vi "Main.vi"(8 "error in":errorcluster, 11 "Pumps Worker in":refnum<class "Pumps Worker.lvclass">) -> (0 "error out":errorcluster, 3 "Pumps Worker out":refnum<class "Pumps Worker.lvclass">)   [LabVIEW 2023, in "pump_Lib.lvlib" / "Pumps Worker.lvclass"]
doc: "The <b>Queued Message Handler</b> of the Worker that owns this VI."
uses:
  Pumps Worker.lvclass
  C:/Program Files/National Instruments/LabVIEW 2023/vi.lib/addons/_Workers/Library/Classes/Worker/Worker.lvclass
  TypeDef/control_Type.ctl
  TypeDef/pump_Type.ctl
  TypeDef/pair_Type.ctl
  Initialization Data.ctl
  Response Cases.ctl
  <vilib>/addons/_Workers/Library/Case Label.ctl
  Pumps Worker.lvclass/Pumps Worker.ctl
  rqp_Stop Session.ctl
  rqp_Get Settings.ctl
  rqp_Write Data.ctl
  TypeDef/pump_Type_Pair_L.ctl
  TypeDef/pump_Type_Pair_R.ctl
  rsp_New Pumps Data.ctl
  <vilib>/Utility/error.llb/Error Cluster From Error Code.vi
  <vilib>/ErrorRing/Error Ring.xnode
  <vilib>/addons/_Workers/Library/Classes/Message Queue/Message Queue.lvclass
  pump_Lib.lvlib
  Workers/Message Pump/Message Pump.lvclass
  <vilib>/addons/_Workers/Library/Workers.lvlib
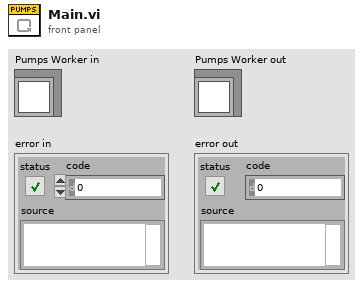
[diagram p1: front panel]
types:
  T1 = typedef "pump_Lib.lvlib/control_Type.ctl" = cluster{"IP Adress in":string, "control_Port_1 ref":refnum<vi>, "control_Port_2 ref":refnum<vi>, "control_Pair ref":refnum<vi>, "queue_Port 1":refnum<queue>, "queue_Port 2":refnum<queue>, "queue_Pair":refnum<queue>, "parametrs ref":refnum<vi>, "Stop Event":refnum<user-event>}
  T2 = typedef "pump_Lib.lvlib/Pumps Worker.lvclass/Initialization Data.ctl" = cluster{"Response Cases":T3}
  T3 = typedef "pump_Lib.lvlib/Pumps Worker.lvclass/Response Cases.ctl" = cluster{"Placeholder - Can be deleted":string, "New Pumps Data":T4}
  T4 = typedef "Workers.lvlib/Case Label.ctl" = string
  T5 = typedef "pump_Lib.lvlib/Pumps Worker.lvclass/rqp_Stop Session.ctl" = cluster{"String":string}
  T6 = typedef "pump_Lib.lvlib/Pumps Worker.lvclass/rqp_Get Settings.ctl" = cluster{"Pump":refnum<vi>, "Params":refnum<vi>, "Pump2":refnum<vi>, "Pump System":refnum<vi>, "IP Adress":string}
  T7 = typedef "pump_Lib.lvlib/Pumps Worker.lvclass/rqp_Write Data.ctl" = cluster{"Насос":T8, "Насос 2":T9, "Насосная система":T10}
  T8 = typedef "pump_Lib.lvlib/pump_Type_Pair_L.ctl" = cluster{"Давление заданное":dbl, "Давление MAX заданное":dbl, "Давление в насосе":dbl, "Давление в системе":dbl, "Расход заданый":dbl, "Расход текущий":dbl, "Объём заданный":dbl, "Объём текущий":dbl, "Позиция насоса %":dbl, "Ток двигателя":dbl, "controlMsg":string, "Клапан k_sys":bool, "Клапан k_res":bool, "Клапан k_air":bool, "Вверх":bool, "Домой":bool, "Вниз":bool, "Старт расход":bool, "Старт давление":bool, "Сброс объёма":bool, "Сброс давления Рсис":bool, "Сброс давления Рнас":bool, "Bits":cluster{"plc_control":bool, "lag_control":bool, "mstop_control":bool, "st_home":bool, "error":bool, "mstart":bool, "pair":bool, "startQ":bool, "startP":bool, "volume_Stop":bool}}
  T9 = typedef "pump_Lib.lvlib/pump_Type_Pair_R.ctl" = cluster{"Давление заданное":dbl, "Давление MAX заданное":dbl, "Давление в насосе":dbl, "Давление в системе":dbl, "Расход заданый":dbl, "Расход текущий":dbl, "Объём заданный":dbl, "Объём текущий":dbl, "Позиция насоса %":dbl, "Ток двигателя":dbl, "controlMsg":string, "Клапан k_sys":bool, "Клапан k_res":bool, "Клапан k_air":bool, "Вверх":bool, "Домой":bool, "Вниз":bool, "Старт расход":bool, "Старт давление":bool, "Сброс объёма":bool, "Сброс давления Рсис":bool, "Сброс давления Рнас":bool, "Bits":cluster{"plc_control":bool, "lag_control":bool, "mstop_control":bool, "st_home":bool, "error":bool, "mstart":bool, "pair":bool, "startQ":bool, "startP":bool, "volume_Stop":bool}}
  T10 = typedef "pump_Lib.lvlib/pair_Type.ctl" = cluster{"Давление заданное":dbl, "Давление в системе":dbl, "Расход заданый":dbl, "Расход текущий":dbl, "Объём заданный":dbl, "Объём текущий":dbl, "Старт давление":bool, "Старт расход":bool, "Сброс объёма":bool, "plc_control":bool, "lag_control":bool, "mstop_control":bool, "Давление":cluster{"АЦП CH 0":dbl, "АЦП CH 1":dbl, "АЦП CH 2":dbl, "АЦП CH 3":dbl, "АЦП CH 4":dbl, "АЦП CH 5":dbl, "АЦП CH 6":dbl, "АЦП CH 7":dbl}, "Modbus":cluster{"Массив чтения":u16[], "Массив записи":u16[]}}
  T11 = typedef "pump_Lib.lvlib/Pumps Worker.lvclass/rsp_New Pumps Data.ctl" = cluster{"Насос":T8, "Насос 2":T9, "Насосная система":T10}
  T12 = typedef "pump_Lib.lvlib/pump_Type.ctl" = cluster{"Давление заданное":dbl, "Давление MAX заданное":dbl, "Давление в насосе":dbl, "Давление в системе":dbl, "Расход заданый":dbl, "Расход текущий":dbl, "Объём заданный":dbl, "Объём текущий":dbl, "Позиция насоса %":dbl, "Ток двигателя":dbl, "controlMsg":string, "Клапан k_sys":bool, "Клапан k_res":bool, "Клапан k_air":bool, "Вверх":bool, "Домой":bool, "Вниз":bool, "Старт расход":bool, "Старт давление":bool, "Сброс объёма":bool, "Сброс давления Рсис":bool, "Сброс давления Рнас":bool, "Bits":cluster{"plc_control":bool, "lag_control":bool, "mstop_control":bool, "st_home":bool, "error":bool, "mstart":bool, "pair":bool, "startQ":bool, "startP":bool, "volume_Stop":bool}}
  T13 = cluster{"IP Adress in":string, "control_Port_1 ref":refnum<vi>, "control_Port_2 ref":refnum<vi>, "control_Pair ref":refnum<vi>, "queue_Port 1":refnum<queue>, "queue_Port 2":refnum<queue>, "queue_Pair":refnum<queue>, "parametrs ref":refnum<vi>, "Stop Event":refnum<user-event>}
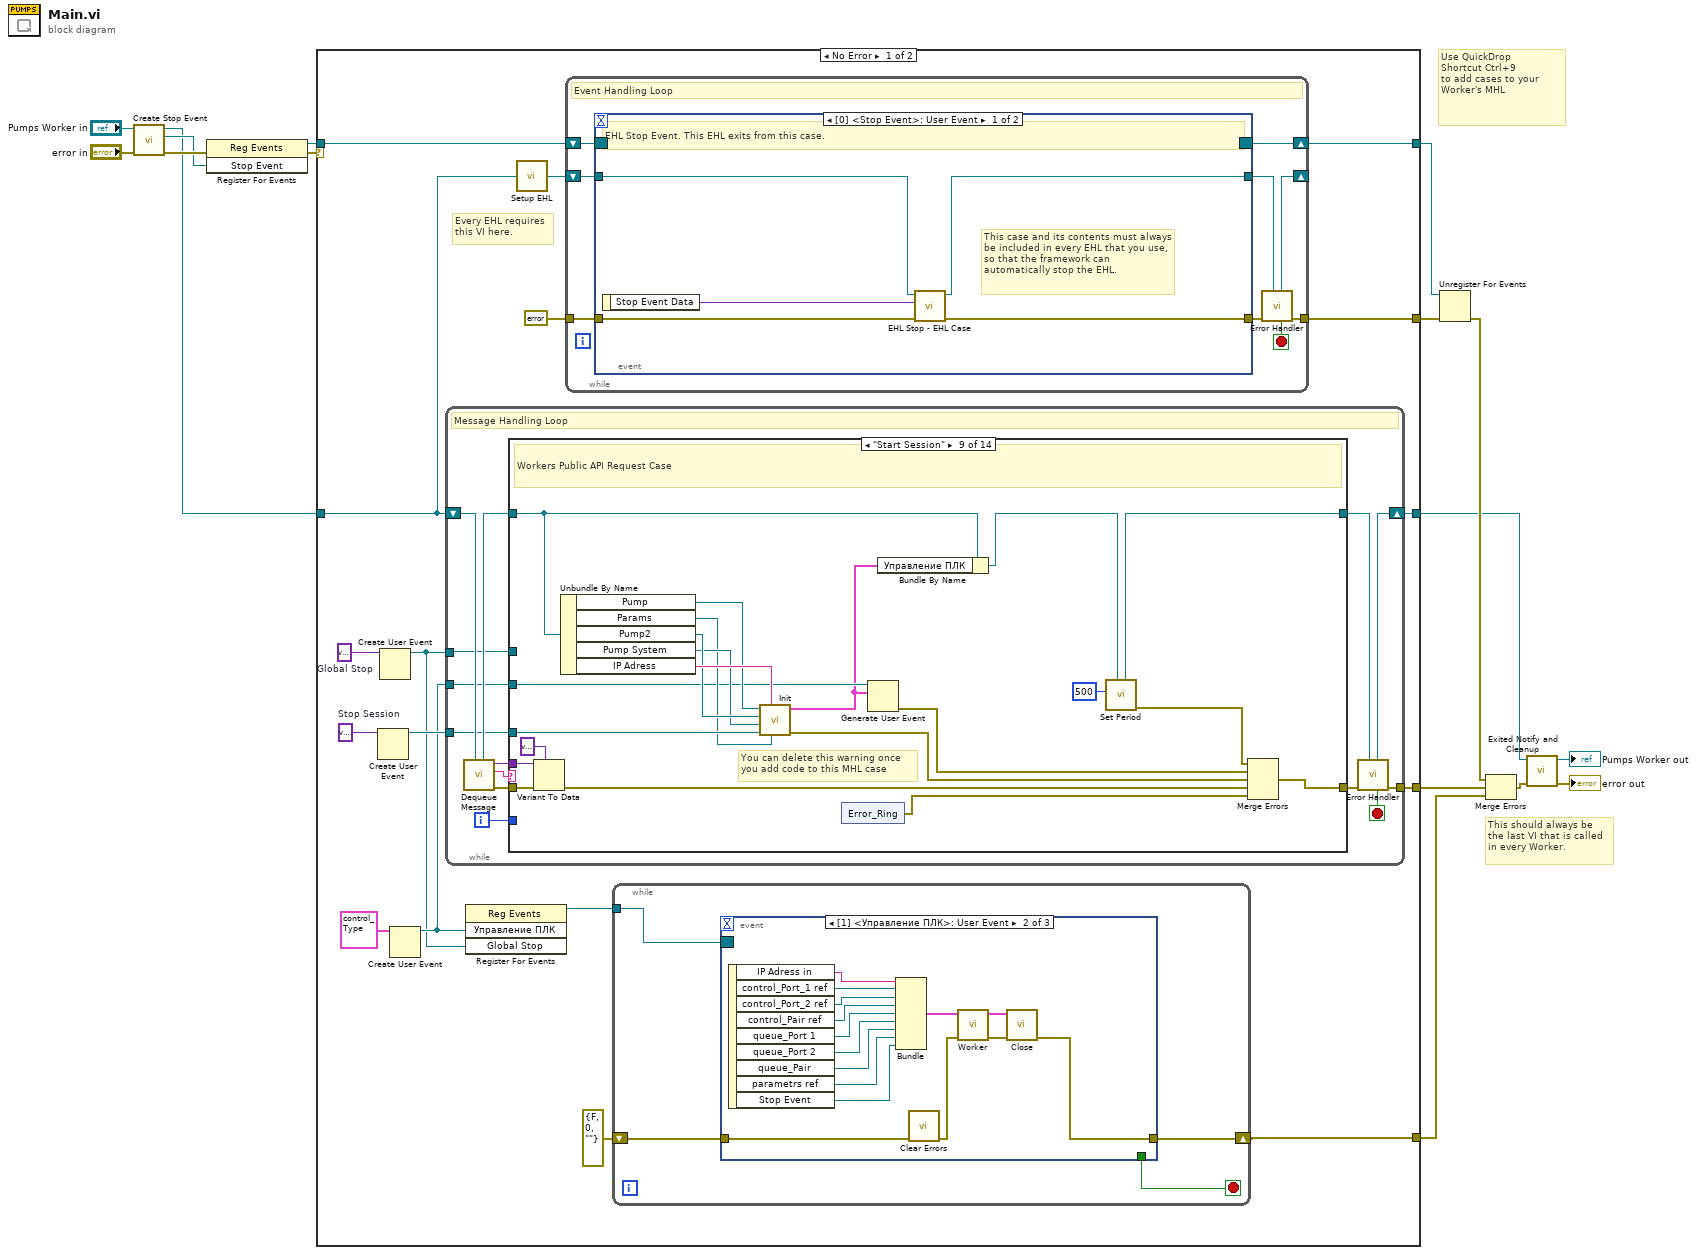
[diagram p0: block diagram]
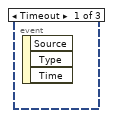
[diagram p2: hidden frame]
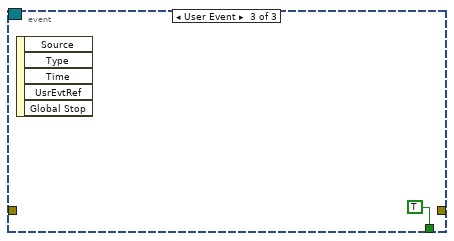
[diagram p3: hidden frame]
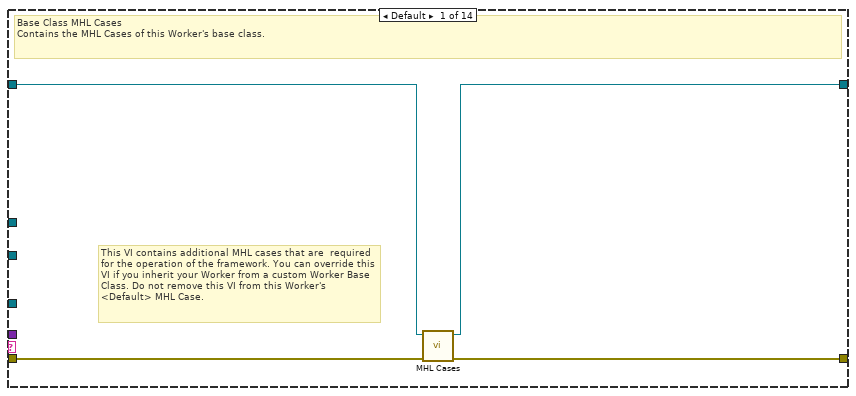
[diagram p4: hidden frame]
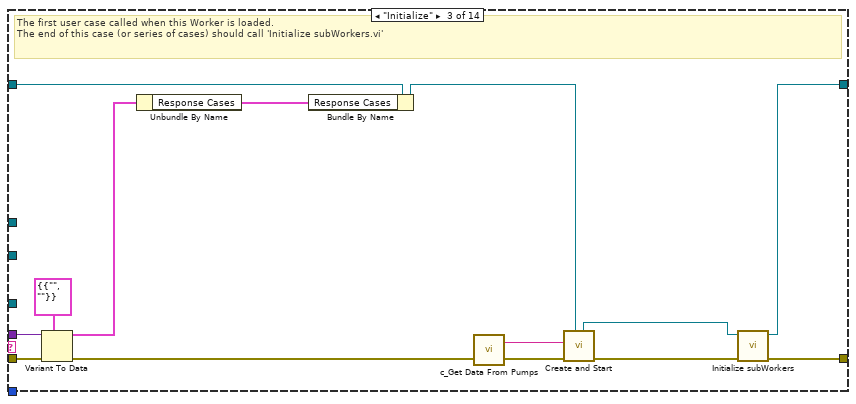
[diagram p6: hidden frame]
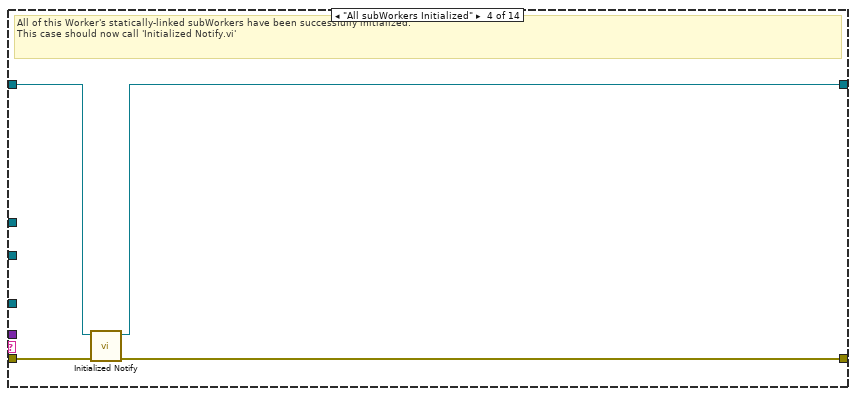
[diagram p7: hidden frame]
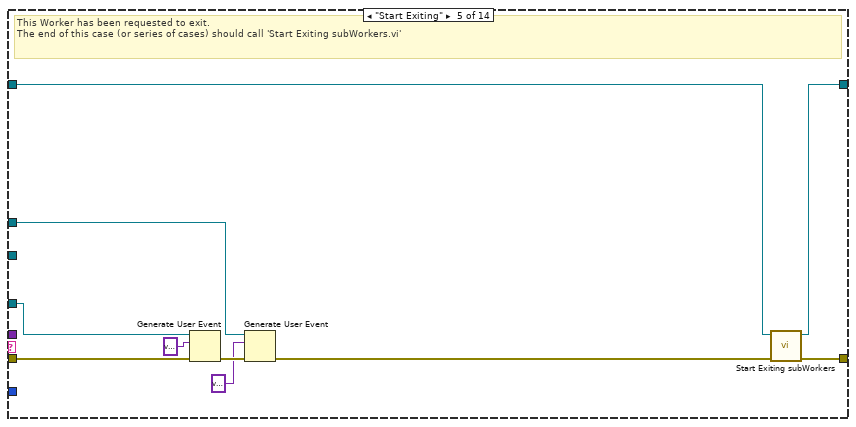
[diagram p8: hidden frame]
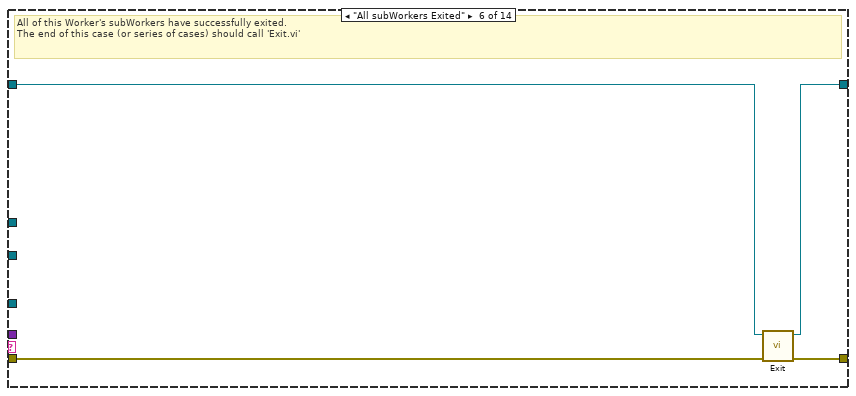
[diagram p9: hidden frame]
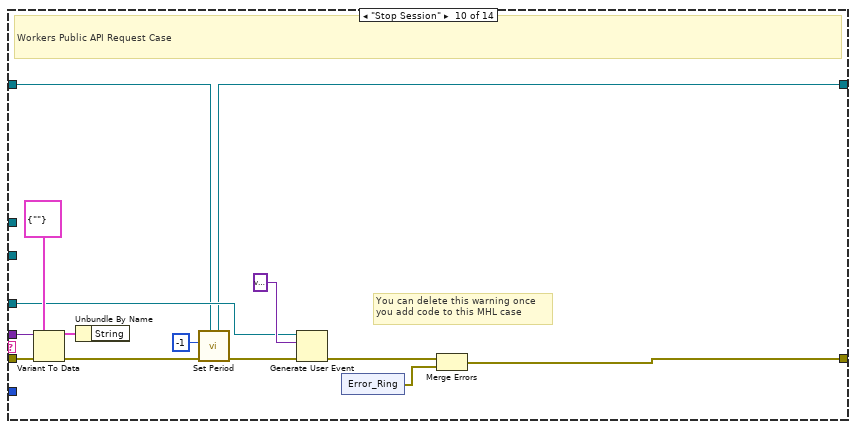
[diagram p12: hidden frame]
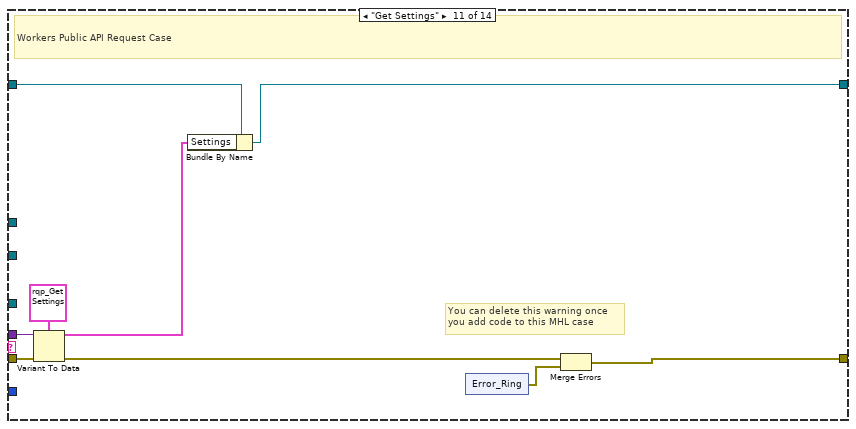
[diagram p13: hidden frame]
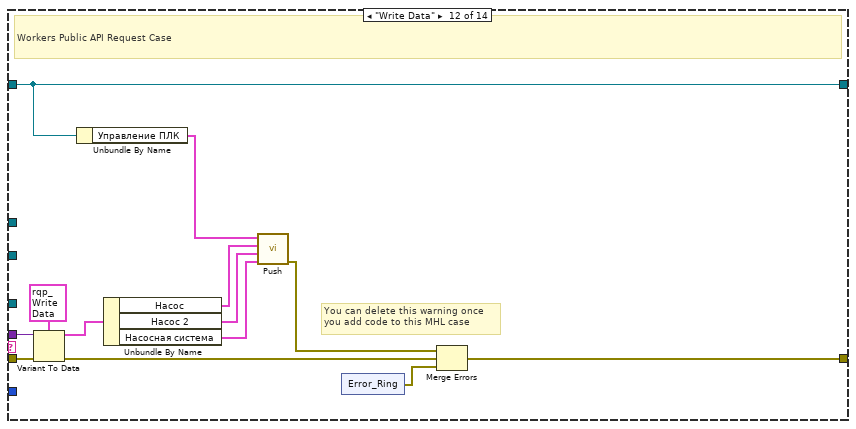
[diagram p14: hidden frame]
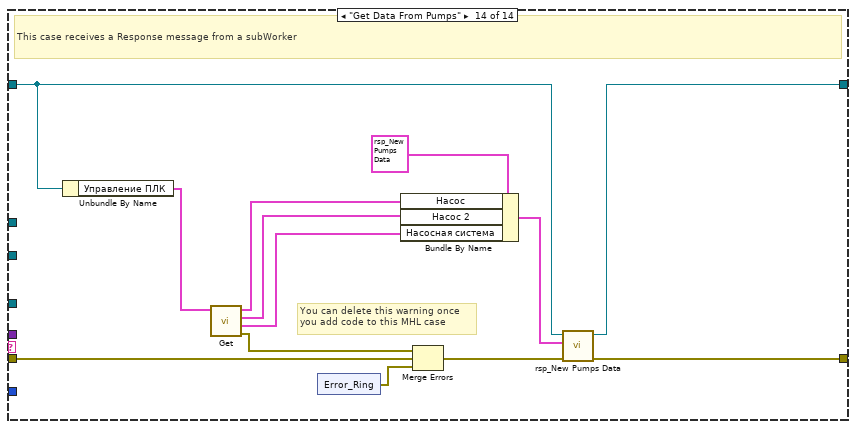
[diagram p16: hidden frame]
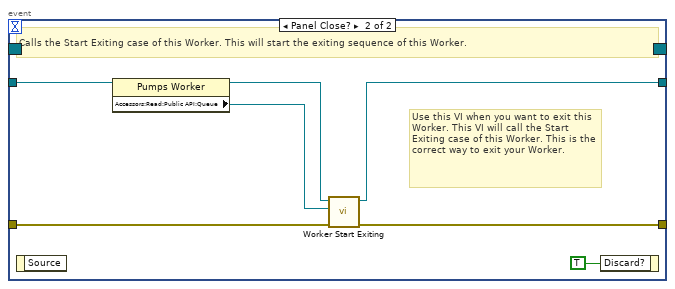
[diagram p17: hidden frame]
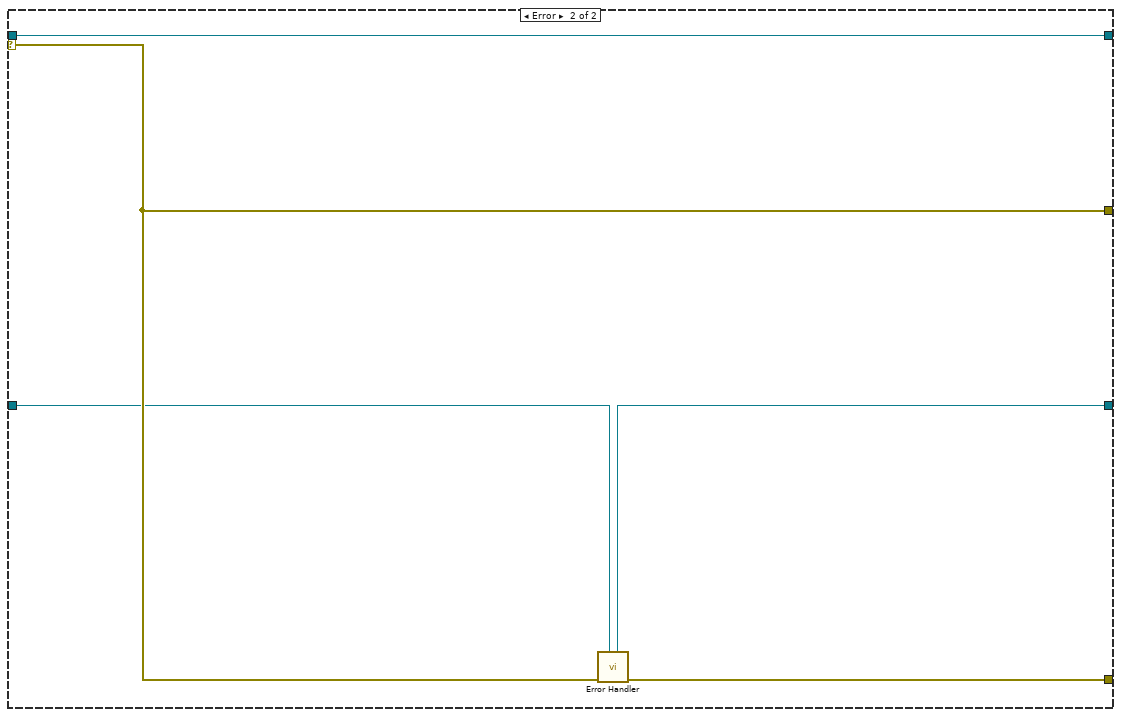
[diagram p18: hidden frame]
diagram:
  # "Use QuickDrop\nShortcut Ctrl+9\nto add cases to your\nWorker's MHL"
  # "This should always be the last VI that is called in every Worker."
  n1 = call-dynamic "Create Stop Event.vi"("error in"="error in", "Worker"="Pumps Worker in") -> ("error out"=w11:errorcluster, "Stop Event"=w8:refnum<user-event>, "Worker out"=w2:refnum<class "Pumps Worker.lvclass">)  [unwired: 7 in]
  n2 = register-events(error in=w11, w8) -> (reference out=w10:refnum<event-registration>, error out=w3:errorcluster)  [unwired: 1 in]
  n3 = case shown="No Error" w3 {
    tunnel: w2 -> [w28 w228]
    tunnel: [w26 w229] -> w9
    tunnel: w10 -> [w33 w230]
    tunnel: [w30 w231] -> w15
    tunnel: [w32 w230] -> w14
    tunnel: [w27 w227] -> w12
    selector: w3 -> [_ w231]
    tunnel: [w18 _] -> w1
    frame No Error {
      w20 = variant  # Global Stop
      w24 = variant  # Stop Session
      # "Every EHL requires\nthis VI here."
      n4 = Create User Event(user event datatype=w24) -> (user event=w23:refnum<user-event>)  [unwired: 1 in, 1 out]
      n5 = Create User Event(user event datatype=w20) -> (user event=w19:refnum<user-event>)  [unwired: 1 in, 1 out]
      n6 = Create User Event(user event datatype=T1 {"IP Adress in"="", "control_Port_1 ref"=refnum, "control_Port_2 ref"=refnum, "control_Pair ref"=refnum, "queue_Port 1"=refnum, "queue_Port 2"=refnum, "queue_Pair"=refnum, "parametrs ref"=refnum, "Stop Event"=refnum} ("Управление ПЛК")) -> (user event=w22:refnum<user-event>)  [unwired: 1 in, 1 out]
      n7 = while {
        shift-right: [w65] -> w27
        shift-left: w28 -> [w67]
        tunnel: [w66] -> w26
        tunnel: w22 -> [w57]
        tunnel: w23 -> [w56]
        tunnel: w19 -> [w54]
        i -> [w58]
        stop <- w59 stop-if-true
        # "Message Handling Loop"
        n8 = call-dynamic "Dequeue Message.vi"("Worker"=w67) -> ("error out"=w64:errorcluster, "Case out"=w60:string, "Data out"=w55:variant, "Worker out"=w62:refnum<class "Pumps Worker.lvclass">)  [unwired: 6 in, 1 out]
        n9 = case "Worker MHL Case Structure (DO NOT CHANGE LABEL NAME)" shown="\"Start Session\"" w60 {
          tunnel: w64 -> [w71 w72 w84 w88 w97 w104 w106 w108 w129 w148 w162 w180 w187 w200]
          tunnel: [w70 w72 w86 w87 w100 w103 w106 w108 w127 w144 w159 w175 w187 w193] -> w63
          tunnel: w62 -> [w69 w73 w83 w90 w98 w102 w105 w107 w115 w136 w157 w169 w186 w196]
          tunnel: [w68 w73 w85 w89 w99 w101 w105 w107 w111 w135 w155 w169 w186 w195] -> w61
          tunnel: w58 -> [_ _ _ _ _ _ _ _ _ _ _ _ _ _]
          tunnel: w57 -> [_ _ _ _ _ _ _ _ w117 _ _ _ _ _]
          tunnel: w56 -> [_ _ _ _ w96 _ _ _ w123 w137 _ _ _ _]
          tunnel: w55 -> [_ _ w82 _ _ _ _ _ w128 w146 w160 w177 _ _]
          tunnel: w54 -> [_ _ _ _ w92 _ _ _ _ _ _ _ _ _]
          frame Default {
            # "This VI contains additional MHL cases that are  required for the operation of the framework. You can override this VI if you inherit your Worker from a custom Worker Base Class. Do not remove this VI from this Worker's <Default> MHL Case."
            # "Base Class MHL Cases\nContains the MHL Cases of this Worker's base class."
            n10 = call-dynamic "MHL Cases.vi"("error in"=w71, "Worker in"=w69) -> ("error out"=w70:errorcluster, "Worker out"=w68:refnum<class "Pumps Worker.lvclass">)  [unwired: 8 in]
          }
          frame "------------ FRAMEWORK CASES -----------" {
            # "Start of Workers Framework Cases"
          }
          frame "Initialize" {
            # "The first user case called when this Worker is loaded.\nThe end of this case (or series of cases) should call 'Initialize subWorkers.vi'"
            n11 = Variant To Data(error in=w84, type=T2 {"Response Cases"={"Placeholder - Can be deleted"="", "New Pumps Data"=""}} ("Initialization Data"), Variant=w82) -> (data=w81:T2, error out=w75:errorcluster)
            n12 = Unbundle By Name(w81) -> ("Response Cases"=w80:T3)
            n13 = Bundle By Name(cluster=w83, "Response Cases"=w80) -> (w77:refnum<class "Pumps Worker.lvclass">)
            n14 = call "c_Get Data From Pumps.vi"() -> ("Case Label"=w78:T4)  [unwired: 1 in]
            n15 = call "Create and Start.vi"("Caller"=w77, "error in (no error)"=w75, "Time Elapsed Response Case (Case Label)"=w78) -> ("error out"=w74:errorcluster, "dup Caller out"=w76:refnum<class "Pumps Worker.lvclass">)  [unwired: 6 in, 1 out]
            n16 = call-dynamic "Initialize subWorkers.vi"("error in"=w74, "Worker"=w76) -> ("error out"=w86:errorcluster, "dup Worker out"=w85:refnum<class "Pumps Worker.lvclass">)  [unwired: 8 in]
          }
          frame "All subWorkers Initialized" {
            # "All of this Worker's statically-linked subWorkers have been successfully initialized.\nThis case should now call 'Initialized Notify.vi'"
            n17 = call-dynamic "Initialized Notify.vi"("error in"=w88, "Worker"=w90) -> ("error out"=w87:errorcluster, "dup Worker out"=w89:refnum<class "Pumps Worker.lvclass">)  [unwired: 8 in]
          }
          frame "Start Exiting" {
            # "This Worker has been requested to exit. \nThe end of this case (or series of cases) should call 'Start Exiting subWorkers.vi'"
            n18 = Generate User Event(user event=w96, event data cluster=variant ("event data"), error in=w97) -> (error out=w94:errorcluster)  [unwired: 1 in, 1 out]
            n19 = Generate User Event(user event=w92, event data cluster=variant ("event data"), error in=w94) -> (error out=w93:errorcluster)  [unwired: 1 in, 1 out]
            n20 = call-dynamic "Start Exiting subWorkers.vi"("error_in"=w93, "Worker"=w98) -> ("error out"=w100:errorcluster, "dup Worker out"=w99:refnum<class "Pumps Worker.lvclass">)  [unwired: 8 in]
          }
          frame "All subWorkers Exited" {
            # "All of this Worker's subWorkers have successfully exited. \nThe end of this case (or series of cases) should call 'Exit.vi'"
            n21 = call-dynamic "Exit.vi"("error_in"=w104, "Worker"=w102) -> ("error out"=w103:errorcluster, "dup Worker out"=w101:refnum<class "Pumps Worker.lvclass">)  [unwired: 8 in]
          }
          frame "------------- LOCAL API CASES -------------" {
            # "Start of Workers Local API Cases"
          }
          frame "------------- PUBLIC API CASES -------------" {
            # "Start of Workers Public API Cases"
          }
          frame "Start Session" {
            # "You can delete this warning once\nyou add code to this MHL case"
            # "Workers Public API Request Case"
            n22 = Variant To Data(error in=w129, type=variant, Variant=w128) -> (error out=w125:errorcluster)  [unwired: 1 out]
            n23 = Unbundle By Name(w115) -> ("Pump"=w121:refnum<vi>, "Params"=w118:refnum<vi>, "Pump2"=w120:refnum<vi>, "Pump System"=w119:refnum<vi>, "IP Adress"=w122:string)
            n24 = call "Init.vi"("parametrs ref"=w118, "IP Adress in"=w122, "Stop Event"=w123, "control_Pair ref"=w119, "control_Port_2 ref"=w120, "control_Port_1 ref"=w121) -> ("error out"=w124:errorcluster, "Управление ПЛК"=w114:T1)  [unwired: 4 in]
            n25 = xnode ("Error_Ring")() -> ("error out"=w126:errorcluster)
            n26 = Generate User Event(user event=w117, event data cluster=w114) -> (error out=w116:errorcluster)  [unwired: 2 in, 1 out]
            n27 = Bundle By Name(cluster=w115, "Управление ПЛК"=w114) -> (w112:refnum<class "Pumps Worker.lvclass">)
            n28 = call "Set Period.vi"("Caller"=w112, "Period (ms)"=500) -> ("error out"=w110:errorcluster, "dup Caller out"=w111:refnum<class "Pumps Worker.lvclass">)  [unwired: 8 in]
            n29 = Merge Errors(w110, w116, w124, w125, w126) -> (w127:errorcluster)
          }
          frame "Stop Session" {
            # "You can delete this warning once\nyou add code to this MHL case"
            # "Workers Public API Request Case"
            n30 = Variant To Data(error in=w148, type=T5 {"String"=""} ("Data"), Variant=w146) -> (data=w145:T5, error out=w139:errorcluster)
            n31 = Unbundle By Name(w145) -> ()  [unwired: 1 out]
            n32 = call "Set Period.vi"("Caller"=w136, "error in"=w139, "Period (ms)"=-1) -> ("error out"=w138:errorcluster, "dup Caller out"=w135:refnum<class "Pumps Worker.lvclass">)  [unwired: 7 in]
            n33 = Generate User Event(user event=w137, event data cluster=variant ("event data"), error in=w138) -> (error out=w142:errorcluster)  [unwired: 1 in, 1 out]
            n34 = xnode ("Error_Ring")() -> ("error out"=w143:errorcluster)
            n35 = Merge Errors(w142, w143) -> (w144:errorcluster)
          }
          frame "Get Settings" {
            # "You can delete this warning once\nyou add code to this MHL case"
            # "Workers Public API Request Case"
            n36 = Variant To Data(error in=w162, type=T6 {"Pump"=refnum, "Params"=refnum, "Pump2"=refnum, "Pump System"=refnum, "IP Adress"=""} ("Data"), Variant=w160) -> (data=w156:T6, error out=w154:errorcluster)
            n37 = Bundle By Name(cluster=w157, "Settings"=w156) -> (w155:refnum<class "Pumps Worker.lvclass">)
            n38 = xnode ("Error_Ring")() -> ("error out"=w158:errorcluster)
            n39 = Merge Errors(w154, w158) -> (w159:errorcluster)
          }
          frame "Write Data" {
            # "You can delete this warning once\nyou add code to this MHL case"
            # "Workers Public API Request Case"
            n40 = Variant To Data(error in=w180, type=T7 {"Насос"={"Давление заданное"=0.3, "Давление MAX заданное"=100.0, "Давление в насосе"=0.0, "Давление в системе"=99.99, "Расход заданый"=0.0, "Расход текущий"=0.0, "Объём заданный"=0.0, "Объём текущий"=0.0, "Позиция насоса %"=0.0, "Ток двигателя"=0.0, "controlMsg"="", "Клапан k_sys"=FALSE, "Клапан k_res"=FALSE, "Клапан k_air"=FALSE, "Вверх"=FALSE, "Домой"=FALSE, "Вниз"=FALSE, "Старт расход"=FALSE, "Старт давление"=FALSE, "Сброс объёма"=FALSE, "Сброс давления Рсис"=FALSE, "Сброс давления Рнас"=FALSE, "Bits"={"plc_control"=FALSE, "lag_control"=FALSE, "mstop_control"=FALSE, "st_home"=FALSE, "error"=FALSE, "mstart"=FALSE, "pair"=FALSE, "startQ"=FALSE, "startP"=FALSE, "volume_Stop"=FALSE}}, "Насос 2"={"Давление заданное"=0.3, "Давление MAX заданное"=100.0, "Давление в насосе"=0.0, "Давление в системе"=99.99, "Расход заданый"=0.0, "Расход текущий"=0.0, "Объём заданный"=0.0, "Объём текущий"=0.0, "Позиция насоса %"=0.0, "Ток двигателя"=0.0, "controlMsg"="", "Клапан k_sys"=FALSE, "Клапан k_res"=FALSE, "Клапан k_air"=FALSE, "Вверх"=FALSE, "Домой"=FALSE, "Вниз"=FALSE, "Старт расход"=FALSE, "Старт давление"=FALSE, "Сброс объёма"=FALSE, "Сброс давления Рсис"=FALSE, "Сброс давления Рнас"=FALSE, "Bits"={"plc_control"=FALSE, "lag_control"=FALSE, "mstop_control"=FALSE, "st_home"=FALSE, "error"=FALSE, "mstart"=FALSE, "pair"=FALSE, "startQ"=FALSE, "startP"=FALSE, "volume_Stop"=FALSE}}, "Насосная система"={"Давление заданное"=0.3, "Давление в системе"=99.99, "Расход заданый"=0.0, "Расход текущий"=0.0, "Объём заданный"=0.0, "Объём текущий"=0.0, "Старт давление"=FALSE, "Старт расход"=FALSE, "Сброс объёма"=FALSE, "plc_control"=FALSE, "lag_control"=FALSE, "mstop_control"=FALSE, "Давление"={"АЦП CH 0"=0.0, "АЦП CH 1"=0.0, "АЦП CH 2"=0.0, "АЦП CH 3"=0.0, "АЦП CH 4"=0.0, "АЦП CH 5"=0.0, "АЦП CH 6"=0.0, "АЦП CH 7"=0.0}, "Modbus"={"Массив чтения"=[], "Массив записи"=[]}}} ("Data"), Variant=w177) -> (data=w176:T7, error out=w179:errorcluster)
            n41 = Unbundle By Name(w169) -> ("Управление ПЛК"=w168:T1)
            n42 = Unbundle By Name(w176) -> ("Насос"=w172:T8, "Насос 2"=w171:T9, "Насосная система"=w170:T10)
            n43 = call "Push.vi"("Pair in"=w170, "Port 2 in"=w171, "Port 1 in"=w172, "Управление ПЛК"=w168) -> ("error out"=w173:errorcluster)  [unwired: 4 in, 3 out]
            n44 = xnode ("Error_Ring")() -> ("error out"=w174:errorcluster)
            n45 = Merge Errors(w173, w179, w174) -> (w175:errorcluster)
          }
          frame "------------- RESPONSE CASES --------------" {
            # "Start of Workers Response Cases"
          }
          frame "Get Data From Pumps" {
            # "You can delete this warning once\nyou add code to this MHL case"
            # "This case receives a Response message from a subWorker"
            n46 = Unbundle By Name(w196) -> ("Управление ПЛК"=w197:T1)
            n47 = call "Get.vi"("Управление ПЛК"=w197) -> ("error out"=w198:errorcluster, "Pair out"=w189:T10, "Port 2 out"=w190:T12, "Port 1 out"=w191:T12)  [unwired: 7 in]
            n48 = xnode ("Error_Ring")() -> ("error out"=w199:errorcluster)
            n49 = Bundle By Name(cluster=T11 {"Насос"={"Давление заданное"=0.3, "Давление MAX заданное"=100.0, "Давление в насосе"=0.0, "Давление в системе"=99.99, "Расход заданый"=0.0, "Расход текущий"=0.0, "Объём заданный"=0.0, "Объём текущий"=0.0, "Позиция насоса %"=0.0, "Ток двигателя"=0.0, "controlMsg"="", "Клапан k_sys"=FALSE, "Клапан k_res"=FALSE, "Клапан k_air"=FALSE, "Вверх"=FALSE, "Домой"=FALSE, "Вниз"=FALSE, "Старт расход"=FALSE, "Старт давление"=FALSE, "Сброс объёма"=FALSE, "Сброс давления Рсис"=FALSE, "Сброс давления Рнас"=FALSE, "Bits"={"plc_control"=FALSE, "lag_control"=FALSE, "mstop_control"=FALSE, "st_home"=FALSE, "error"=FALSE, "mstart"=FALSE, "pair"=FALSE, "startQ"=FALSE, "startP"=FALSE, "volume_Stop"=FALSE}}, "Насос 2"={"Давление заданное"=0.3, "Давление MAX заданное"=100.0, "Давление в насосе"=0.0, "Давление в системе"=99.99, "Расход заданый"=0.0, "Расход текущий"=0.0, "Объём заданный"=0.0, "Объём текущий"=0.0, "Позиция насоса %"=0.0, "Ток двигателя"=0.0, "controlMsg"="", "Клапан k_sys"=FALSE, "Клапан k_res"=FALSE, "Клапан k_air"=FALSE, "Вверх"=FALSE, "Домой"=FALSE, "Вниз"=FALSE, "Старт расход"=FALSE, "Старт давление"=FALSE, "Сброс объёма"=FALSE, "Сброс давления Рсис"=FALSE, "Сброс давления Рнас"=FALSE, "Bits"={"plc_control"=FALSE, "lag_control"=FALSE, "mstop_control"=FALSE, "st_home"=FALSE, "error"=FALSE, "mstart"=FALSE, "pair"=FALSE, "startQ"=FALSE, "startP"=FALSE, "volume_Stop"=FALSE}}, "Насосная система"={"Давление заданное"=0.3, "Давление в системе"=99.99, "Расход заданый"=0.0, "Расход текущий"=0.0, "Объём заданный"=0.0, "Объём текущий"=0.0, "Старт давление"=FALSE, "Старт расход"=FALSE, "Сброс объёма"=FALSE, "plc_control"=FALSE, "lag_control"=FALSE, "mstop_control"=FALSE, "Давление"={"АЦП CH 0"=0.0, "АЦП CH 1"=0.0, "АЦП CH 2"=0.0, "АЦП CH 3"=0.0, "АЦП CH 4"=0.0, "АЦП CH 5"=0.0, "АЦП CH 6"=0.0, "АЦП CH 7"=0.0}, "Modbus"={"Массив чтения"=[], "Массив записи"=[]}}} ("Data in"), "Насос"=w191, "Насос 2"=w190, "Насосная система"=w189) -> (w188:T11)
            n50 = Merge Errors(w198, w200, w199) -> (w194:errorcluster)
            n51 = call "rsp_New Pumps Data.vi"("error in"=w194, "Data in"=w188, "Pumps Worker in"=w196) -> ("error out"=w193:errorcluster, "dup Pumps Worker out"=w195:refnum<class "Pumps Worker.lvclass">)  [unwired: 7 in]
          }
        }
        n52 = call-dynamic "Error Handler.vi"("Worker"=w61, "error_in"=w63) -> ("error out"=w66:errorcluster, "Stop Loop"=w59:bool, "Worker out"=w65:refnum<class "Pumps Worker.lvclass">)  [unwired: 7 in]
      }
      n53 = register-events(w22, w19) -> (reference out=w25:refnum<event-registration>)  [unwired: 2 in, 1 out]
      n54 = call-dynamic "Setup EHL.vi"("Worker"=w28) -> ("Worker out"=w29:refnum<class "Pumps Worker.lvclass">)  [unwired: 14 in]
      n55 = while "Event Handling Loop" {
        shift-right: [w214] -> w32
        shift-left: w33 -> [w213]
        tunnel: [w209] -> w30
        tunnel: errorcluster {"status"=FALSE, "code"=0, "source"=""} ("error constant") -> [w211]
        shift-right: [w207] -> _
        shift-left: w29 -> [w212]
        stop <- w206 stop-if-true
        # "Event Handling Loop"
        n56 = event shown="[0] <Stop Event>: User Event" {
          selector: w213 -> [_ _]
          dyn-events: [_ _] -> w214
          timeout: _ -> [_ _]
          tunnel: [w218 w225] -> w210
          tunnel: w211 -> [w219 w224]
          tunnel: w212 -> [w217 w223]
          tunnel: [w216 w222] -> w208
          event User Event {
            # "This case and its contents must always be included in every EHL that you use, so that the framework can automatically stop the EHL."
            # "EHL Stop Event. This EHL exits from this case."
            n57 = event-data() -> ("Stop Event Data"=w215:variant)  [unwired: 1 in]
            n58 = call-dynamic "EHL Stop - EHL Case.vi"("error in"=w219, "Stop Event Data"=w215, "Worker"=w217) -> ("error out"=w218:errorcluster, "Worker out"=w216:refnum<class "Pumps Worker.lvclass">)  [unwired: 7 in]
          }
          event Panel Close? {
            # "Use this VI when you want to exit this Worker. This VI will call the Start Exiting case of this Worker. This is the correct way to exit your Worker."
            # "Calls the Start Exiting case of this Worker. This will start the exiting sequence of this Worker."
            n59 = event-data() -> ()  [unwired: 1 in, 1 out]
            n60 = property class="Pumps Worker"(reference=w223) -> (reference out=w221:refnum<class "Pumps Worker.lvclass">, "Accessors:Read:Public API:Queue"=w220:refnum<class "Message Queue.lvclass">)  [unwired: 1 in, 1 out]
            n61 = call-dynamic "Worker Start Exiting.vi"("error_in"=w224, "Message Queue"=w220, "Worker"=w221) -> ("error out"=w225:errorcluster, "dup Worker out"=w222:refnum<class "Pumps Worker.lvclass">)  [unwired: 7 in]
            n62 = event-data("Discard?"=TRUE) -> ()  [unwired: 1 in, 1 out]
          }
        }
        n63 = call-dynamic "Error Handler.vi"("Worker"=w208, "error_in"=w210) -> ("error out"=w209:errorcluster, "Stop Loop"=w206:bool, "Worker out"=w207:refnum<class "Pumps Worker.lvclass">)  [unwired: 7 in]
      }
      n64 = while {
        tunnel: w25 -> [w37]
        shift-right: [w35] -> w18
        shift-left: errorcluster {"status"=FALSE, "code"=0, "source"=""} ("Error Out") -> [w34]
        stop <- w36 stop-if-true
        n65 = event shown="[1] <Управление ПЛК>: User Event" {
          selector: w37 -> [_ _ _]
          dyn-events: _ -> [_ _ _]
          timeout: _ -> [_ _ _]
          tunnel: [_ _ TRUE] -> w36
          tunnel: [_ w38 _] -> w35
          tunnel: w34 -> [_ w42 _]
          event Timeout {
            n66 = event-data() -> ()  [unwired: 1 in, 3 out]
          }
          event User Event {
            n67 = event-data() -> ("IP Adress in"=w52:string, "control_Port_1 ref"=w51:refnum<vi>, "control_Port_2 ref"=w50:refnum<vi>, "control_Pair ref"=w49:refnum<vi>, "queue_Port 1"=w48:refnum<queue>, "queue_Port 2"=w47:refnum<queue>, "queue_Pair"=w46:refnum<queue>, "parametrs ref"=w45:refnum<vi>, "Stop Event"=w44:refnum<user-event>)  [unwired: 1 in]
            n68 = Bundle("IP Adress in"=w52, "control_Port_1 ref"=w51, "control_Port_2 ref"=w50, "control_Pair ref"=w49, "queue_Port 1"=w48, "queue_Port 2"=w47, "queue_Pair"=w46, "parametrs ref"=w45, "Stop Event"=w44) -> (w43:T13)  [unwired: 1 in]
            n69 = call <vilib>:"Clear Errors.vi"("error in (no error)"=w42) -> ("error out"=w41:errorcluster)  [unwired: 5 in, 1 out]
            n70 = call "Worker.vi"("Error In"=w41, "Управление ПЛК вход"=w43) -> ("Error Out"=w39:errorcluster, "Управление ПЛК выход"=w40:T1)  [unwired: 8 in]
            n71 = call "Close.vi"("Error In"=w39, "Управление ПЛК"=w40) -> ("error out"=w38:errorcluster)  [unwired: 9 in]
          }
          event User Event {
            n72 = event-data() -> ()  [unwired: 1 in, 5 out]
          }
        }
      }
    }
    frame Error {
      n73 = call-dynamic "Error Handler.vi"("Worker"=w228, "error_in"=w231) -> ("error out"=w229:errorcluster, "Worker out"=w227:refnum<class "Pumps Worker.lvclass">)  [unwired: 7 in, 1 out]
    }
  }
  n74 = Unregister For Events(event registration refnum=w14, error in=w15) -> (error out=w16:errorcluster)
  n75 = Merge Errors(w16, w9, w1) -> (w13:errorcluster)
  n76 = call-dynamic "Exited Notify and Cleanup.vi"("error_in"=w13, "Worker"=w12) -> ("error out"=→"error out":errorcluster, "dup Worker out"=→"Pumps Worker out":refnum<class "Pumps Worker.lvclass">)  [unwired: 8 in]
